vi "Wago Chamber Control Variables AO.vi"(8 "error in (no error)":errorcluster, 10 "Wago Data Input":T2 {"Input Process Image"."Software Constants"."Room PID Settings"."Room Dehumid Temperature I (*RM Dehum I1)" max=30000 step=1; "Input Process Image"."Software Constants"."Room PID Settings"."Room Dehumid Temperature P (*RM Dehum P1)" max=30000 step=1; "Input Process Image"."Software Constants"."Room PID Settings"."Room Cool Temperature I (*RM Cool I1)" max=30000 step=1; "Input Process Image"."Software Constants"."Room PID Settings"."Room Cool Temperature P (*RM Cool P1)" max=30000 step=1; "Input Process Image"."Software Constants"."Room PID Settings"."Room Heat I (*RM Heat I1)" max=30000 step=1; "Input Process Image"."Software Constants"."Room PID Settings"."Room Heat P (*RM Heat P1)" max=30000 step=1; "Input Process Image"."Software Constants"."Room PID Settings"."Room Humidity I (*RM Hum I1)" max=30000 step=1; "Input Process Image"."Software Constants"."Room PID Settings"."Room Humidity P (*RM Hum P1)" max=30000 step=1; "Input Process Image"."Software Constants"."Room PID Settings"."Room Dry I (*RM Dry I1)" max=30000 step=1; "Input Process Image"."Software Constants"."Room PID Settings"."Room Dry P(*RM Dry P1)" max=30000 step=1}, 11 "Modbus Master in":refnum<class "Modbus Master.lvclass">) -> (0 "error out":errorcluster, 2 "Wago Data Output":T2 {"Input Process Image"."Software Constants"."Room PID Settings"."Room Dehumid Temperature I (*RM Dehum I1)" max=30000 step=1; "Input Process Image"."Software Constants"."Room PID Settings"."Room Dehumid Temperature P (*RM Dehum P1)" max=30000 step=1; "Input Process Image"."Software Constants"."Room PID Settings"."Room Cool Temperature I (*RM Cool I1)" max=30000 step=1; "Input Process Image"."Software Constants"."Room PID Settings"."Room Cool Temperature P (*RM Cool P1)" max=30000 step=1; "Input Process Image"."Software Constants"."Room PID Settings"."Room Heat I (*RM Heat I1)" max=30000 step=1; "Input Process Image"."Software Constants"."Room PID Settings"."Room Heat P (*RM Heat P1)" max=30000 step=1; "Input Process Image"."Software Constants"."Room PID Settings"."Room Humidity I (*RM Hum I1)" max=30000 step=1; "Input Process Image"."Software Constants"."Room PID Settings"."Room Humidity P (*RM Hum P1)" max=30000 step=1; "Input Process Image"."Software Constants"."Room PID Settings"."Room Dry I (*RM Dry I1)" max=30000 step=1; "Input Process Image"."Software Constants"."Room PID Settings"."Room Dry P(*RM Dry P1)" max=30000 step=1}, 3 "Modbus Master out":refnum<class "Modbus Master.lvclass">)   [LabVIEW 2016]
uses:
  <vilib>/NI/Modbus Library/API/Master/Modbus Master.lvclass
  Type Definitions/Wago Main Control.ctl
  Type Definitions/Wago Output Data Process Image.ctl
  Type Definitions/Wago Room Condtions.ctl
  Type Definitions/Wago Door Relays.ctl
  Type Definitions/Wago Contactor Settings.ctl
  Type Definitions/Wago Ground Leakage.ctl
  Type Definitions/Wago Input Process Image.ctl
  Type Definitions/Wago Room PID Settings.ctl
  Type Definitions/Wago Measured Input Data.ctl
  Type Definitions/Wago Room Setpoint Targets.ctl
  Type Definitions/Wago Output Commands.ctl
panel:
  in  "Wago Output Words 4":T1=512 items=["twHeatCtrl"=512, "twSteamCtrl"=513, "twCoolCtrl"=514, "twDehumCtrl"=515, "Output QX4 Bool"=516, "Output QX5 Bool"=517, "Output QX6 Bool"=518, "Output QX7 Bool"=519, "Output QX8 Bool"=520, "Output QX9 Bool"=521, "Output QX10"=522, "twRoomTemp"=840, "twRoomHum"=841, "twSuppTemp"=842, "twCoolTemp"=843, "twDehumTemp"=844, "twGlycolTemp"=845, "twHeatRate"=846, "twSteamRate"=847, "twCoolRate"=848, "twDehumRate"=849, "twStatus"=850, "twDoorEna"=851, "Rm1St1Dr1Stat"=816, "Rm1St2Dr1Stat"=817, "Rm1St3Dr1Stat"=818, "Rm1St4Dr1Stat"=819, "Rm1St5Dr1Stat"=820, "Rm1St6Dr1Stat"=821, "Rm1St7Dr1Stat"=822, "Rm1St8Dr1Stat"=823, "Rm1St1Dr2Stat"=824, "Rm1St2Dr2Stat"=825, "Rm1St3Dr2Stat"=826, "Rm1St4Dr2Stat"=827, "Rm1St5Dr2Stat"=828, "Rm1St6DrStat"=829, "Rm1St7Dr2Stat"=830, "Rm1St8Dr2Stat"=831, "Rm1St1Dr3Stat"=832, "Rm1St2Dr3Stat"=833, "Rm1St3Dr3Stat"=834, "Rm1St4Dr3Stat"=835, "Rm1St5Dr3Stat"=836, "Rm1St6Dr3Stat"=837, "Rm1St7Dr3Stat"=838, "Rm1St8Dr3Stat"=839, "twVoltMon1"=784, "twVoltMon2"=785, "twVoltMon3"=786, "twVoltMon4"=787, "twVoltMon5"=788, "twVoltMon6"=789, "twVoltMon7"=790, "twVoltMon8"=791, "twVoltStat1"=792, "twVoltStat2"=793, "twVoltStat3"=794, "twVoltStat4"=795, "twVoltStat5"=796, "twVoltStat6"=797, "twVoltStat7"=798, "twVoltStat8"=799]
  in  "Wago Output Words 3":T1=513 items=["twHeatCtrl"=512, "twSteamCtrl"=513, "twCoolCtrl"=514, "twDehumCtrl"=515, "Output QX4 Bool"=516, "Output QX5 Bool"=517, "Output QX6 Bool"=518, "Output QX7 Bool"=519, "Output QX8 Bool"=520, "Output QX9 Bool"=521, "Output QX10"=522, "twRoomTemp"=840, "twRoomHum"=841, "twSuppTemp"=842, "twCoolTemp"=843, "twDehumTemp"=844, "twGlycolTemp"=845, "twHeatRate"=846, "twSteamRate"=847, "twCoolRate"=848, "twDehumRate"=849, "twStatus"=850, "twDoorEna"=851, "Rm1St1Dr1Stat"=816, "Rm1St2Dr1Stat"=817, "Rm1St3Dr1Stat"=818, "Rm1St4Dr1Stat"=819, "Rm1St5Dr1Stat"=820, "Rm1St6Dr1Stat"=821, "Rm1St7Dr1Stat"=822, "Rm1St8Dr1Stat"=823, "Rm1St1Dr2Stat"=824, "Rm1St2Dr2Stat"=825, "Rm1St3Dr2Stat"=826, "Rm1St4Dr2Stat"=827, "Rm1St5Dr2Stat"=828, "Rm1St6DrStat"=829, "Rm1St7Dr2Stat"=830, "Rm1St8Dr2Stat"=831, "Rm1St1Dr3Stat"=832, "Rm1St2Dr3Stat"=833, "Rm1St3Dr3Stat"=834, "Rm1St4Dr3Stat"=835, "Rm1St5Dr3Stat"=836, "Rm1St6Dr3Stat"=837, "Rm1St7Dr3Stat"=838, "Rm1St8Dr3Stat"=839, "twVoltMon1"=784, "twVoltMon2"=785, "twVoltMon3"=786, "twVoltMon4"=787, "twVoltMon5"=788, "twVoltMon6"=789, "twVoltMon7"=790, "twVoltMon8"=791, "twVoltStat1"=792, "twVoltStat2"=793, "twVoltStat3"=794, "twVoltStat4"=795, "twVoltStat5"=796, "twVoltStat6"=797, "twVoltStat7"=798, "twVoltStat8"=799]
  in  "Wago Output Words 2":T1=514 items=["twHeatCtrl"=512, "twSteamCtrl"=513, "twCoolCtrl"=514, "twDehumCtrl"=515, "Output QX4 Bool"=516, "Output QX5 Bool"=517, "Output QX6 Bool"=518, "Output QX7 Bool"=519, "Output QX8 Bool"=520, "Output QX9 Bool"=521, "Output QX10"=522, "twRoomTemp"=840, "twRoomHum"=841, "twSuppTemp"=842, "twCoolTemp"=843, "twDehumTemp"=844, "twGlycolTemp"=845, "twHeatRate"=846, "twSteamRate"=847, "twCoolRate"=848, "twDehumRate"=849, "twStatus"=850, "twDoorEna"=851, "Rm1St1Dr1Stat"=816, "Rm1St2Dr1Stat"=817, "Rm1St3Dr1Stat"=818, "Rm1St4Dr1Stat"=819, "Rm1St5Dr1Stat"=820, "Rm1St6Dr1Stat"=821, "Rm1St7Dr1Stat"=822, "Rm1St8Dr1Stat"=823, "Rm1St1Dr2Stat"=824, "Rm1St2Dr2Stat"=825, "Rm1St3Dr2Stat"=826, "Rm1St4Dr2Stat"=827, "Rm1St5Dr2Stat"=828, "Rm1St6DrStat"=829, "Rm1St7Dr2Stat"=830, "Rm1St8Dr2Stat"=831, "Rm1St1Dr3Stat"=832, "Rm1St2Dr3Stat"=833, "Rm1St3Dr3Stat"=834, "Rm1St4Dr3Stat"=835, "Rm1St5Dr3Stat"=836, "Rm1St6Dr3Stat"=837, "Rm1St7Dr3Stat"=838, "Rm1St8Dr3Stat"=839, "twVoltMon1"=784, "twVoltMon2"=785, "twVoltMon3"=786, "twVoltMon4"=787, "twVoltMon5"=788, "twVoltMon6"=789, "twVoltMon7"=790, "twVoltMon8"=791, "twVoltStat1"=792, "twVoltStat2"=793, "twVoltStat3"=794, "twVoltStat4"=795, "twVoltStat5"=796, "twVoltStat6"=797, "twVoltStat7"=798, "twVoltStat8"=799]
  in  "Wago Output Words":T1=515 items=["twHeatCtrl"=512, "twSteamCtrl"=513, "twCoolCtrl"=514, "twDehumCtrl"=515, "Output QX4 Bool"=516, "Output QX5 Bool"=517, "Output QX6 Bool"=518, "Output QX7 Bool"=519, "Output QX8 Bool"=520, "Output QX9 Bool"=521, "Output QX10"=522, "twRoomTemp"=840, "twRoomHum"=841, "twSuppTemp"=842, "twCoolTemp"=843, "twDehumTemp"=844, "twGlycolTemp"=845, "twHeatRate"=846, "twSteamRate"=847, "twCoolRate"=848, "twDehumRate"=849, "twStatus"=850, "twDoorEna"=851, "Rm1St1Dr1Stat"=816, "Rm1St2Dr1Stat"=817, "Rm1St3Dr1Stat"=818, "Rm1St4Dr1Stat"=819, "Rm1St5Dr1Stat"=820, "Rm1St6Dr1Stat"=821, "Rm1St7Dr1Stat"=822, "Rm1St8Dr1Stat"=823, "Rm1St1Dr2Stat"=824, "Rm1St2Dr2Stat"=825, "Rm1St3Dr2Stat"=826, "Rm1St4Dr2Stat"=827, "Rm1St5Dr2Stat"=828, "Rm1St6DrStat"=829, "Rm1St7Dr2Stat"=830, "Rm1St8Dr2Stat"=831, "Rm1St1Dr3Stat"=832, "Rm1St2Dr3Stat"=833, "Rm1St3Dr3Stat"=834, "Rm1St4Dr3Stat"=835, "Rm1St5Dr3Stat"=836, "Rm1St6Dr3Stat"=837, "Rm1St7Dr3Stat"=838, "Rm1St8Dr3Stat"=839, "twVoltMon1"=784, "twVoltMon2"=785, "twVoltMon3"=786, "twVoltMon4"=787, "twVoltMon5"=788, "twVoltMon6"=789, "twVoltMon7"=790, "twVoltMon8"=791, "twVoltStat1"=792, "twVoltStat2"=793, "twVoltStat3"=794, "twVoltStat4"=795, "twVoltStat5"=796, "twVoltStat6"=797, "twVoltStat7"=798, "twVoltStat8"=799]
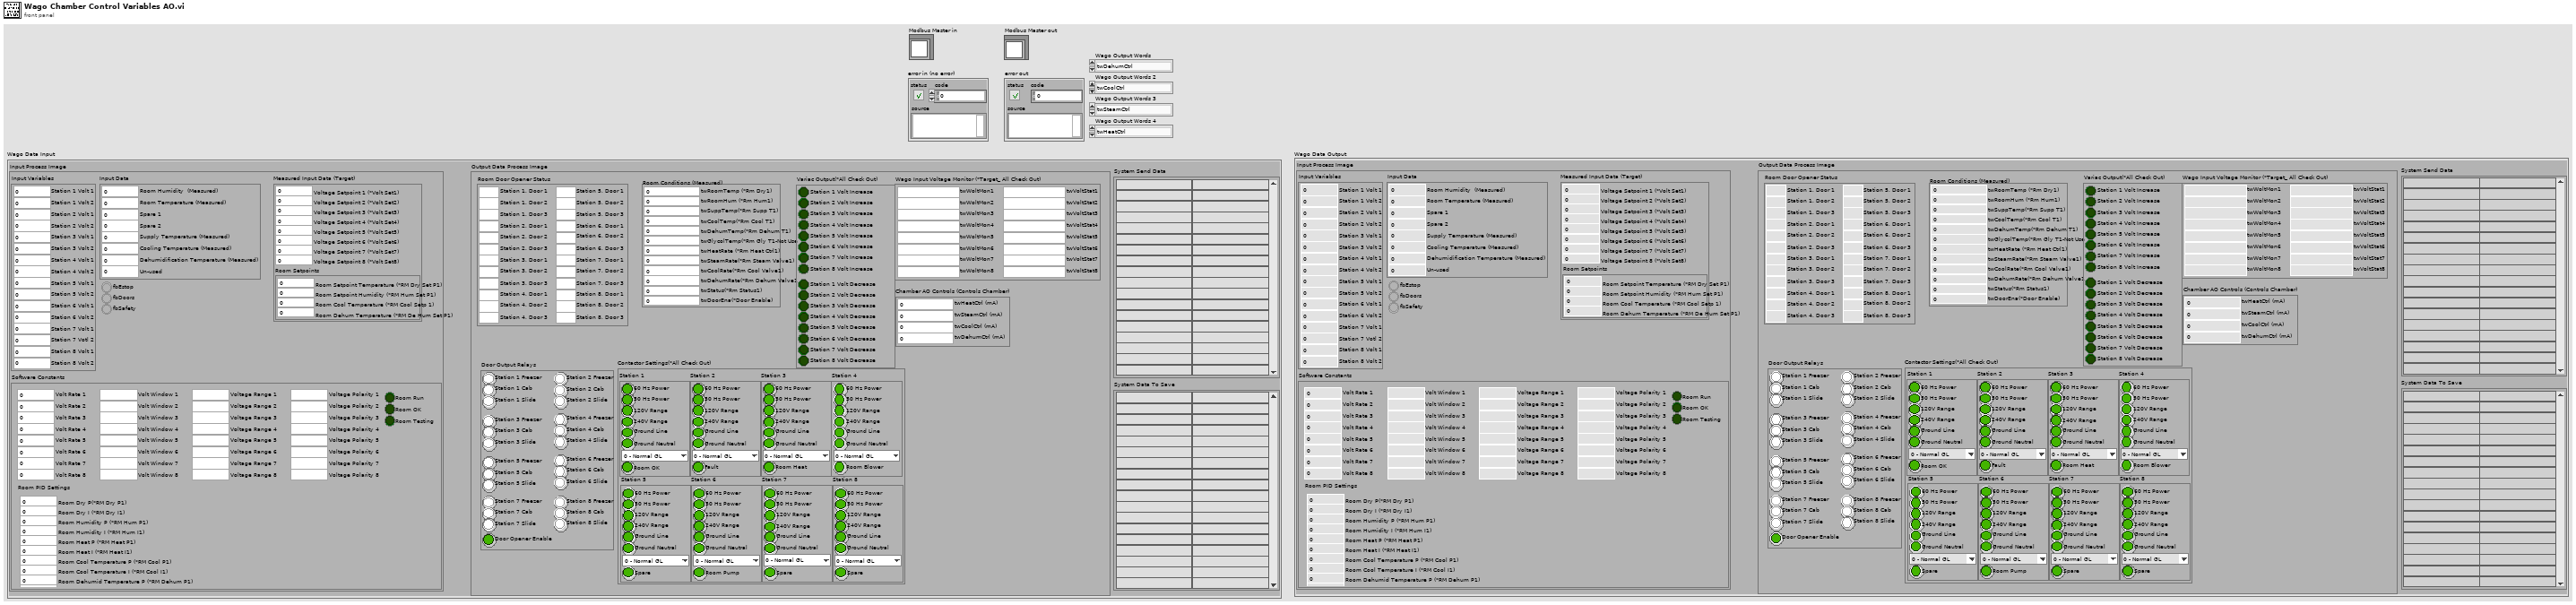
[diagram p1: front panel]
types:
  T1 = typedef "Wago Output Commands.ctl" = u16
  T2 = typedef "Wago Main Control.ctl" = cluster{"Output Data Process Image":T3, "Input Process Image":T8, "System Send Data":string[][], "System Data To Save":string[][]}
  T3 = typedef "Wago Output Data Process Image.ctl" = cluster{"Room Door Opener Status":cluster{"Station 1, Door 1":u16, "Station 1, Door 2":u16, "Station 1, Door 3":u16, "Station 2, Door 1":u16, "Station 2, Door 2":u16, "Station 2, Door 3":u16, "Station 3, Door 1":u16, "Station 3, Door 2":u16, "Station 3, Door 3":u16, "Station 4, Door 1":u16, "Station 4, Door 2":u16, "Station 4, Door 3":u16, "Station 5, Door 1":u16, "Station 5, Door 2":u16, "Station 5, Door 3":u16, "Station 6, Door 1":u16, "Station 6, Door 2":u16, "Station 6, Door 3":u16, "Station 7, Door 1":u16, "Station 7, Door 2":u16, "Station 7, Door 3":u16, "Station 8, Door 1":u16, "Station 8, Door 2":u16, "Station 8, Door 3":u16}, "Room Conditions (Measured)":T4, "Chamber AO Controls (Controls Chamber)":cluster{"twDehumCtrl (mA)":u16, "twCoolCtrl (mA)":u16, "twSteamCtrl (mA)":u16, "twHeatCtrl (mA)":u16}, "Variac Output(*All Check Out)":cluster{"Station 1 Volt Increase":bool, "Station 1 Volt Decrease":bool, "Station 2 Volt Increase":bool, "Station 2 Volt Decrease":bool, "Station 3 Volt Increase":bool, "Station 3 Volt Decrease":bool, "Station 4 Volt Increase":bool, "Station 4 Volt Decrease":bool, "Station 5 Volt Increase":bool, "Station 5 Volt Decrease":bool, "Station 6 Volt Increase":bool, "Station 6 Volt Decrease":bool, "Station 7 Volt Increase":bool, "Station 7 Volt Decrease":bool, "Station 8 Volt Increase":bool, "Station 8 Volt Decrease":bool}, "Door Output Relays":T5, "Wago Input Voltage Monitor (*Target_ All Check Out)":cluster{"twWoltMon1":dbl, "twWoltMon2":dbl, "twWoltMon3":dbl, "twWoltMon4":dbl, "twWoltMon5":dbl, "twWoltMon6":dbl, "twWoltMon7":dbl, "twWoltMon8":dbl, "twVoltStat1":u16, "twVoltStat2":u16, "twVoltStat3":u16, "twVoltStat4":u16, "twVoltStat5":u16, "twVoltStat6":u16, "twVoltStat7":u16, "twVoltStat8":u16}, "Contactor Settings(*All Check Out)":T6}
  T4 = typedef "Wago Room Condtions.ctl" = cluster{"twDoorEna(*Door Enable)":u16, "twStatus(*Rm Status1)":u16, "twRoomTemp (*Rm Dry1)":dbl, "twRoomHum (*Rm Hum1)":dbl, "twSuppTemp(*Rm Supp T1)":dbl, "twCoolTemp(*Rm Cool T1)":dbl, "twDehumTemp(*Rm Dehum T1)":dbl, "twGlycolTemp(*Rm Gly T1-Not Used)":dbl, "twDehumRate(*Rm Dehum Valve1)":dbl, "twCoolRate(*Rm Cool Valve1)":dbl, "twSteamRate(*Rm Steam Valve1)":dbl, "twHeatRate (*Rm Heat Ctrl1)":dbl}
  T5 = typedef "Wago Door Relays.ctl" = cluster{"Station 1 Freezer":bool, "Station 1 Cab":bool, "Station 1 Slide":bool, "Station 2 Freezer":bool, "Station 2 Cab":bool, "Station 2 Slide":bool, "Station 3 Freezer":bool, "Station 3 Cab":bool, "Station 3 Slide":bool, "Station 4 Freezer":bool, "Station 4 Cab":bool, "Station 4 Slide":bool, "Station 5 Freezer":bool, "Station 5 Cab":bool, "Station 5 Slide":bool, "Station 6 Freezer":bool, "Station 6 Cab":bool, "Station 6 Slide":bool, "Station 7 Freezer":bool, "Station 7 Cab":bool, "Station 7 Slide":bool, "Station 8 Freezer":bool, "Station 8 Cab":bool, "Station 8 Slide":bool, "Door Opener Enable":bool}
  T6 = typedef "Wago Contactor Settings.ctl" = cluster{"Station 1":cluster{"60 Hz Power":bool, "50 Hz Power":bool, "120V Range":bool, "240V Range":bool, "Ground Line":bool, "Ground Neutral":bool, "Room OK":bool, "Ground Leakage":T7}, "Station 2":cluster{"60 Hz Power":bool, "50 Hz Power":bool, "120V Range":bool, "240V Range":bool, "Ground Line":bool, "Ground Neutral":bool, "Fault":bool, "Ground Leakage":T7}, "Station 3":cluster{"60 Hz Power":bool, "50 Hz Power":bool, "120V Range":bool, "240V Range":bool, "Ground Line":bool, "Ground Neutral":bool, "Room Heat":bool, "Ground Leakage":T7}, "Station 4":cluster{"60 Hz Power":bool, "50 Hz Power":bool, "120V Range":bool, "240V Range":bool, "Ground Line":bool, "Ground Neutral":bool, "Room Blower":bool, "Ground Leakage":T7}, "Station 5":cluster{"60 Hz Power":bool, "50 Hz Power":bool, "120V Range":bool, "240V Range":bool, "Ground Line":bool, "Ground Neutral":bool, "Spare":bool, "Ground Leakage":T7}, "Station 6":cluster{"60 Hz Power":bool, "50 Hz Power":bool, "120V Range":bool, "240V Range":bool, "Ground Line":bool, "Ground Neutral":bool, "Room Pump":bool, "Ground Leakage":T7}, "Station 7":cluster{"60 Hz Power":bool, "50 Hz Power":bool, "120V Range":bool, "240V Range":bool, "Ground Line":bool, "Ground Neutral":bool, "Spare":bool, "Ground Leakage":T7}, "Station 8":cluster{"60 Hz Power":bool, "50 Hz Power":bool, "120V Range":bool, "240V Range":bool, "Ground Line":bool, "Ground Neutral":bool, "Spare":bool, "Ground Leakage":T7}}
  T7 = typedef "Wago Ground Leakage.ctl" = enum16{"0 - Normal GL", "1 - Measure GL"}
  T8 = typedef "Wago Input Process Image.ctl" = cluster{"fbEstop":bool, "fbDoors":bool, "fbSafety":bool, "Input Variables":cluster{"Station 1 Volt 1":dbl, "Station 1 Volt 2":dbl, "Station 2 Volt 1":dbl, "Station 2 Volt 2":dbl, "Station 3 Volt 1":dbl, "Station 3 Volt 2":dbl, "Station 4 Volt 1":dbl, "Station 4 Volt 2":dbl, "Station 5 Volt 1":dbl, "Station 5 Volt 2":dbl, "Station 6 Volt 1":dbl, "Station 6 Volt 2":dbl, "Station 7 Volt 1":dbl, "Station 7 Votl 2":dbl, "Station 8 Volt 1":dbl, "Station 8 Volt 2":dbl}, "Input Data":cluster{"Room Humidity  (Measured)":dbl, "Room Temperature (Measured)":dbl, "Spare 1":dbl, "Spare 2":dbl, "Supply Temperature (Measured)":dbl, "Cooling Temperature (Measured)":dbl, "Dehumidification Temperature (Measured)":dbl, "Un-used":dbl}, "Software Constants":cluster{"Volt Rate 1":u16, "Volt Rate 2":u16, "Volt Rate 3":u16, "Volt Rate 4":u16, "Volt Rate 5":u16, "Volt Rate 6":u16, "Volt Rate 7":u16, "Volt Rate 8":u16, "Volt Window 1":u16, "Volt Window 2":u16, "Volt Window 3":u16, "Volt Window 4":u16, "Volt Window 5":u16, "Volt Window 6":u16, "Volt Window 7":u16, "Volt Window 8":u16, "Voltage Range 1":u16, "Voltage Range 2":u16, "Voltage Range 3":u16, "Voltage Range 4":u16, "Voltage Range 5":u16, "Voltage Range 6":u16, "Voltage Range 7":u16, "Voltage Range 8":u16, "Voltage Polarity 1":u16, "Voltage Polarity 2":u16, "Voltage Polarity 3":u16, "Voltage Polarity 4":u16, "Voltage Polarity 5":u16, "Voltage Polarity 6":u16, "Voltage Polarity 7":u16, "Voltage Polarity 8":u16, "Room Run":bool, "Room OK":bool, "Room Testing":bool, "Room PID Settings":T9}, "Measured Input Data (Target)":T10}
  T9 = typedef "Wago Room PID Settings.ctl" = cluster{"Room Dry P(*RM Dry P1)":u16, "Room Dry I (*RM Dry I1)":u16, "Room Humidity P (*RM Hum P1)":u16, "Room Humidity I (*RM Hum I1)":u16, "Room Heat P (*RM Heat P1)":u16, "Room Heat I (*RM Heat I1)":u16, "Room Cool Temperature P (*RM Cool P1)":u16, "Room Cool Temperature I (*RM Cool I1)":u16, "Room Dehumid Temperature P (*RM Dehum P1)":u16, "Room Dehumid Temperature I (*RM Dehum I1)":u16}
  T10 = typedef "Wago Measured Input Data.ctl" = cluster{"Voltage Setpoint 1 (*Volt Set1)":dbl, "Voltage Setpoint 2 (*Volt Set2)":dbl, "Voltage Setpoint 3 (*Volt Set3)":dbl, "Voltage Setpoint 4 (*Volt Set4)":dbl, "Voltage Setpoint 5 (*Volt Set5)":dbl, "Voltage Setpoint 6 (*Volt Set6)":dbl, "Voltage Setpoint 7 (*Volt Set7)":dbl, "Voltage Setpoint 8 (*Volt Set8)":dbl, "Room Setpoints":T11}
  T11 = typedef "Wago Room Setpoint Targets.ctl" = cluster{"Room Setpoint Temperature (*RM Dry Set P1)":dbl, "Room Setpoint Humidity (*RM Hum Set P1)":dbl, "Room Cool Temperature (*RM Cool Setp 1)":dbl, "Room Dehum Temperature (*RM De Hum Set P1)":dbl}
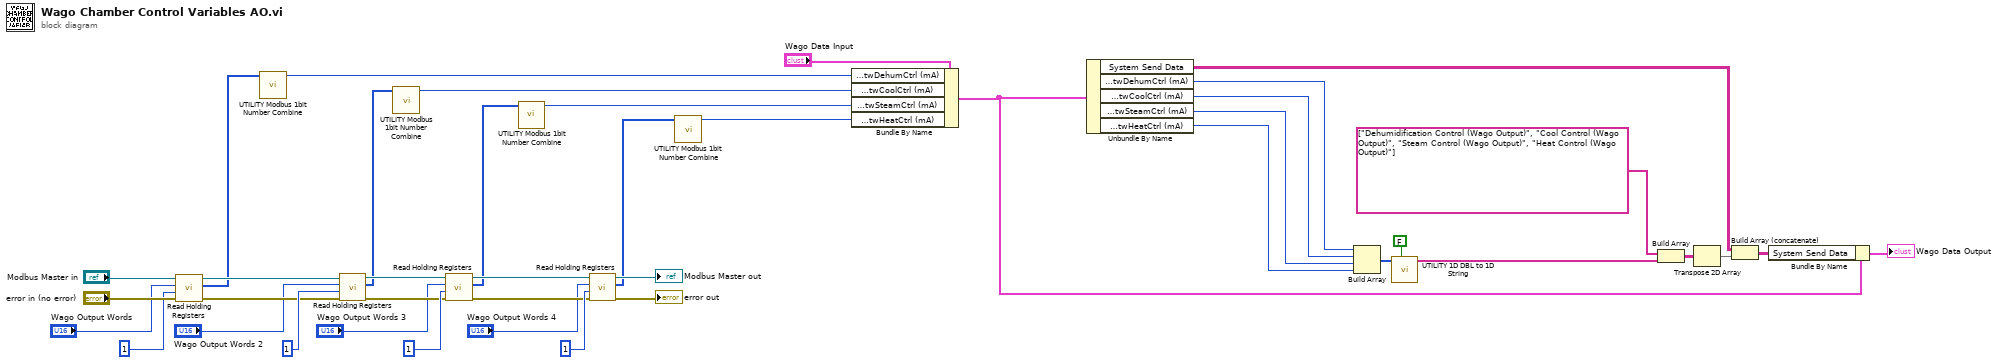
[diagram p0: block diagram]
diagram:
  n1 = call-dynamic "Read Holding Registers.vi"("error in"="error in (no error)", "number of inputs"=u16 1 ("Quantity"), "starting address"="Wago Output Words", "Modbus master in"="Modbus Master in") -> ("error out"=w31:errorcluster, "register values"=w22:u16[], "Modbus master out"=w32:refnum<class "Modbus Master.lvclass">)  [unwired: 5 in]
  n2 = call "UTILITY Modbus 1bit Number Combine.vi"("register values"=w22) -> ("Data"=w21:u16)  [unwired: 10 in]
  n3 = call-dynamic "Read Holding Registers.vi"("error in"=w31, "number of inputs"=u16 1 ("Quantity"), "starting address"="Wago Output Words 2", "Modbus master in"=w32) -> ("error out"=w34:errorcluster, "register values"=w20:u16[], "Modbus master out"=w35:refnum<class "Modbus Master.lvclass">)  [unwired: 5 in]
  n4 = call "UTILITY Modbus 1bit Number Combine.vi"("register values"=w20) -> ("Data"=w19:u16)  [unwired: 10 in]
  n5 = call-dynamic "Read Holding Registers.vi"("error in"=w34, "number of inputs"=u16 1 ("Quantity"), "starting address"="Wago Output Words 3", "Modbus master in"=w35) -> ("error out"=w37:errorcluster, "register values"=w18:u16[], "Modbus master out"=w38:refnum<class "Modbus Master.lvclass">)  [unwired: 5 in]
  n6 = call "UTILITY Modbus 1bit Number Combine.vi"("register values"=w18) -> ("Data"=w17:u16)  [unwired: 10 in]
  n7 = call-dynamic "Read Holding Registers.vi"("error in"=w37, "number of inputs"=u16 1 ("Quantity"), "starting address"="Wago Output Words 4", "Modbus master in"=w38) -> ("error out"=→"error out":errorcluster, "register values"=w16:u16[], "Modbus master out"=→"Modbus Master out":refnum<class "Modbus Master.lvclass">)  [unwired: 5 in]
  n8 = call "UTILITY Modbus 1bit Number Combine.vi"("register values"=w16) -> ("Data"=w15:u16)  [unwired: 10 in]
  n9 = Bundle By Name(cluster="Wago Data Input", "Output Data Process Image.Chamber AO Controls (Controls Chamber).twDehumCtrl (mA)"=w21, "Output Data Process Image.Chamber AO Controls (Controls Chamber).twCoolCtrl (mA)"=w19, "Output Data Process Image.Chamber AO Controls (Controls Chamber).twSteamCtrl (mA)"=w17, "Output Data Process Image.Chamber AO Controls (Controls Chamber).twHeatCtrl (mA)"=w15) -> (w5:T2)
  n10 = Unbundle By Name(w5) -> ("System Send Data"=w8:string[][], "Output Data Process Image.Chamber AO Controls (Controls Chamber).twDehumCtrl (mA)"=w13:u16, "Output Data Process Image.Chamber AO Controls (Controls Chamber).twCoolCtrl (mA)"=w3:u16, "Output Data Process Image.Chamber AO Controls (Controls Chamber).twSteamCtrl (mA)"=w2:u16, "Output Data Process Image.Chamber AO Controls (Controls Chamber).twHeatCtrl (mA)"=w1:u16)
  n11 = Build Array(w13, w3, w2, w1) -> (w12:u16[])
  n12 = call "UTILITY 1D DBL to 1D String.vi"("DBL?"=FALSE, "1D DBL"=w12) -> ("1D String"=w10:string[])  [unwired: 9 in]
  n13 = Build Array(string[] ["Dehumidification Control (Wago Output)", "Cool Control (Wago Output)", "Steam Control (Wago Output)", "Heat Control (Wago Output)"], w10) -> (w9:string[][])
  n14 = Transpose 2D Array(2D array=w9) -> (transposed array=w7:string[][])
  n15 = Build Array (concatenate)(w8, w7) -> (w6:string[][])
  n16 = Bundle By Name(cluster=w5, "System Send Data"=w6) -> (→"Wago Data Output":T2)
